vi "Tx.vi"(8 "error in (no error)":errorcluster, 10 "Transfer Group in":refnum<class "Transfer Group.lvclass">, 11 "Transceiver Thread in":refnum<class "Transceiver Thread.lvclass">) -> (0 "error out":errorcluster, 2 "Transfer Group out":refnum<class "Transfer Group.lvclass">, 3 "Transceiver Thread out":refnum<class "Transceiver Thread.lvclass">)   [LabVIEW 2017, in "DSF Core.lvlib" / "Transceiver Thread.lvclass"]
uses:
  Transceiver Thread.lvclass
  Transfer Group/Transfer Group.lvclass
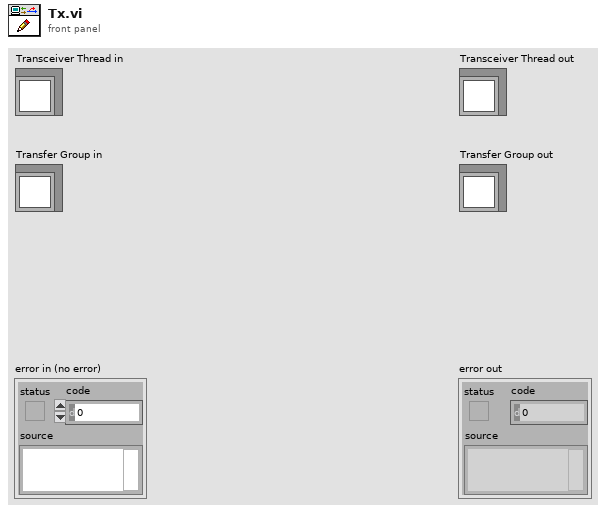
[diagram p1: front panel]
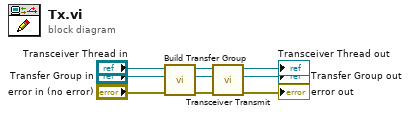
[diagram p0: block diagram]
diagram:
  n1 = call "Build Transfer Group.vi"("error in (no error)"="error in (no error)", "Transfer Group in"="Transfer Group in", "Plugin Thread in"="Transceiver Thread in") -> ("error out"=w8:errorcluster, "Transfer Group out"=w7:refnum<class "Transfer Group.lvclass">, "Plugin Thread out"=w9:refnum<class "Transceiver Thread.lvclass">)  [unwired: 6 in]
  n2 = call "Transceiver Transmit.vi"("error in (no error)"=w8, "Transfer Group in"=w7, "Transceiver Thread in"=w9) -> ("error out"=→"error out":errorcluster, "Transfer Group out"=→"Transfer Group out":refnum<class "Transfer Group.lvclass">, "Transceiver Thread out"=→"Transceiver Thread out":refnum<class "Transceiver Thread.lvclass">)  [unwired: 6 in]
